vi "WFCompose.vi"(7 "Repetitions":T1 {"Interval (s)" min=0.0; "Delay (s)" min=0.0}, 8 "error in (no error)":errorcluster, 11 "Waveform In":waveform(dbl)) -> (0 "error out":errorcluster, 3 "Analog Waveform Out":waveform(dbl))   [LabVIEW 2009]
uses:
  <vilib>/Waveform/WDTOps.llb/WDT Number of Waveform Samples DBL.vi
  <vilib>/Waveform/WDTOps.llb/WDT Waveform Duration DBL.vi
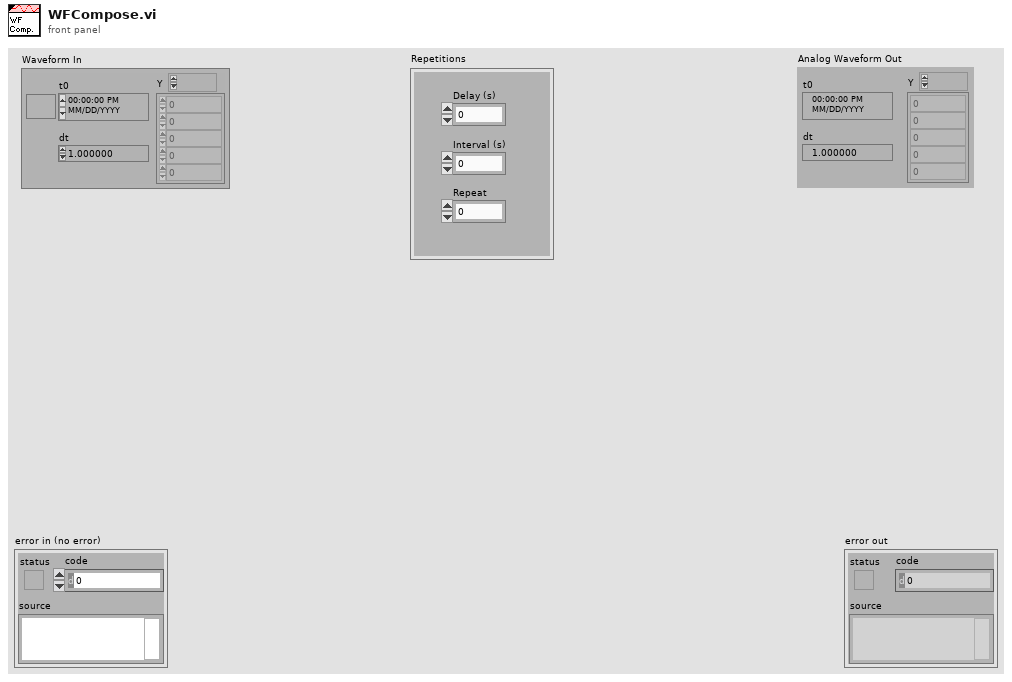
[diagram p1: front panel]
types:
  T1 = cluster{"Delay (s)":dbl, "Interval (s)":dbl, "Repeat":i32}
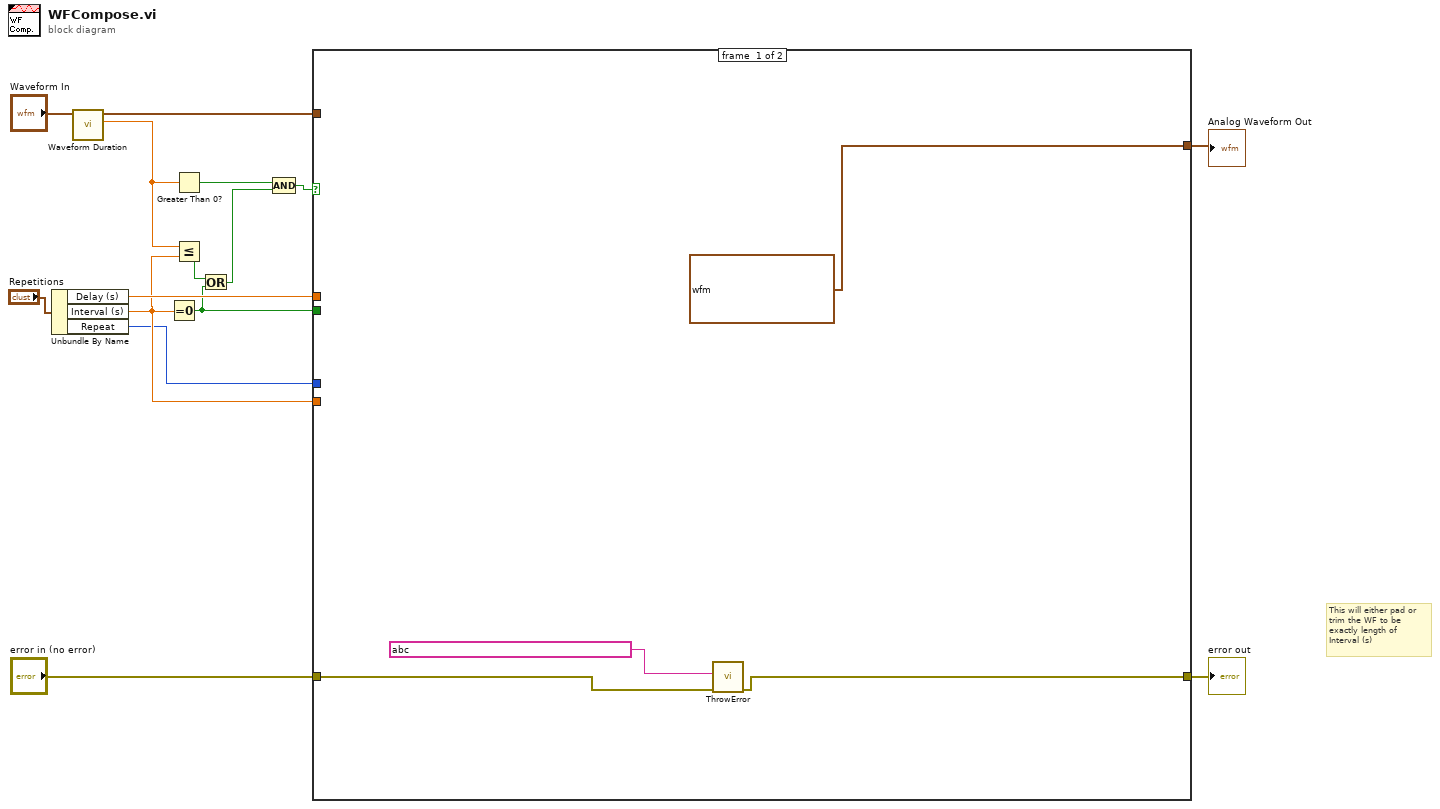
[diagram p0: block diagram]
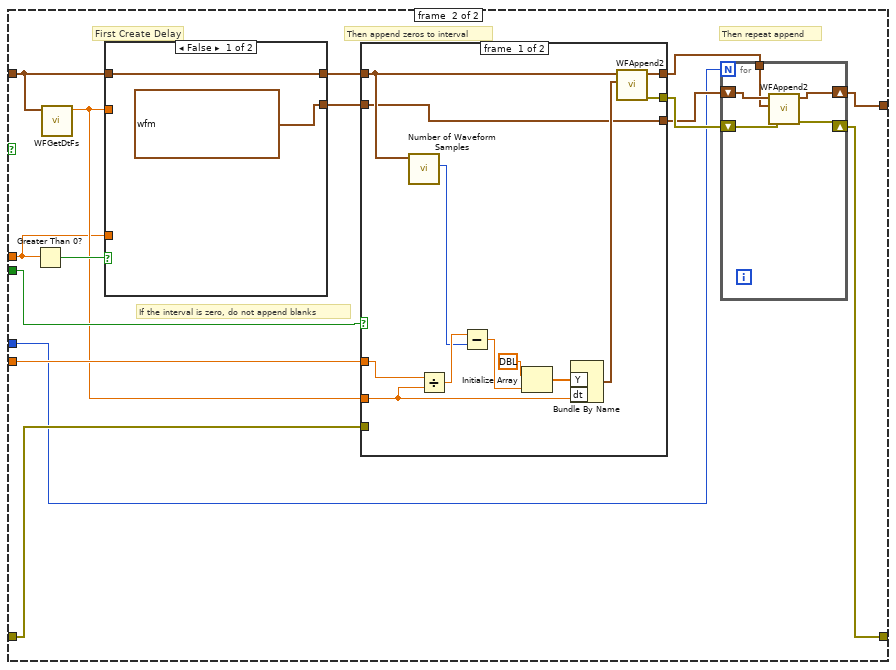
[diagram p2: hidden frame]
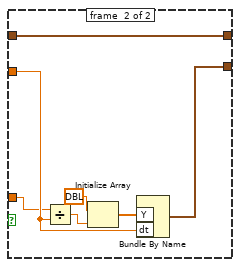
[diagram p4: hidden frame]
diagram:
  # "This will either pad or\ntrim the WF to be\nexactly length of \nInterval (s)"
  n1 = Unbundle By Name("Repetitions") -> ("Delay (s)"=w11:dbl, "Interval (s)"=w7:dbl, "Repeat"=w6:i32)
  n2 = call-poly <vilib>:"Waveform Duration.vi"("waveform in"="Waveform In") -> ("duration"=w5:dbl, "waveform out"=w2:waveform(dbl))  [unwired: 8 in, 1 out]
  n3 = Equal To 0?(x=w7) -> (x = 0?=w1:bool)
  n4 = Greater Than 0?(x=w5) -> (x > 0?=w10:bool)
  n5 = Less Or Equal?(x=w5, y=w7) -> (x <= y?=w12:bool)
  n6 = Or(x=w12, y=w1) -> (x .or. y?=w9:bool)
  n7 = Compound Arithmetic op=AND(w10, w9) -> (w8:bool)
  n8 = case shown="True" w8 {
    tunnel: "error in (no error)" -> [w18 w27]
    tunnel: w2 -> [_ w28]
    tunnel: w11 -> [_ w26]
    tunnel: w1 -> [_ w33]
    tunnel: w7 -> [_ w30]
    tunnel: w6 -> [_ w20]
    tunnel: [waveform(dbl) ? ("Waveform") w25] -> w4
    tunnel: [w17 w24] -> w3
    frame #0 {
      n9 = call "ThrowError.vi"("error in (no error)"=w18, "Error Message"=string ?) -> ("error out"=w17:errorcluster)  [unwired: 8 in, 1 out]
    }
    frame #1 {
      # "Then repeat append"
      # "If the interval is zero, do not append blanks"
      # "First Create Delay"
      # "Then append zeros to interval"
      n10 = Greater Than 0?(x=w26) -> (x > 0?=w34:bool)
      n11 = call "WFGetDtFs.vi"("Waveform"=w28) -> ("dt"=w29:dbl)  [unwired: 9 in, 1 out]
      n12 = case shown="False" w34 {
        tunnel: w28 -> [w56 w59]
        tunnel: [waveform(dbl) ? ("Waveform") w60] -> w32
        tunnel: [w56 w59] -> w31
        tunnel: w29 -> [_ w58]
        tunnel: w26 -> [_ w57]
        frame #0 {
        }
        frame #1 {
          n13 = Divide(x=w57, y=w58) -> (x/y=w61:dbl)
          n14 = Initialize Array(dbl ? ("element"), w61) -> (w63:dbl[])
          n15 = Bundle By Name("Y"=w63, "dt"=w58) -> (w60:waveform(dbl))  [unwired: 1 in]
        }
      }
      n16 = case shown="True" w33 {
        tunnel: w32 -> [w40 w53]
        tunnel: w31 -> [w44 w54]
        tunnel: w30 -> [w49 _]
        tunnel: w29 -> [w48 _]
        tunnel: w27 -> [_ w52]
        tunnel: [w42 w52] -> w23
        tunnel: [w41 w54] -> w22
        tunnel: [w40 w53] -> w21
        frame #0 {
          n17 = call-poly <vilib>:"Number of Waveform Samples.vi"("waveform in"=w44) -> ("number of samples"=w46:i32)  [unwired: 8 in, 2 out]
          n18 = Divide(x=w49, y=w48) -> (x/y=w47:dbl)
          n19 = Subtract(x=w47, y=w46) -> (x-y=w45:dbl)
          n20 = Initialize Array(dbl ? ("element"), w45) -> (w51:dbl[])
          n21 = Bundle By Name("Y"=w51, "dt"=w48) -> (w43:waveform(dbl))  [unwired: 1 in]
          n22 = call "WFAppend2.vi"("Waveform In 2"=w43, "Waveform In"=w44) -> ("error out"=w42:errorcluster, "Waveform Out"=w41:waveform(dbl))  [unwired: 4 in]
        }
        frame #1 {
          # "If interval is zero, just keep appending WF"
        }
      }
      n23 = for {
        N: w20 -> [_]
        shift-right: [w38] -> w25
        shift-left: w21 -> [w39]
        shift-right: [w36] -> w24
        shift-left: w23 -> [w37]
        tunnel: w22 -> [w35]
        n24 = call "WFAppend2.vi"("error in (no error)"=w37, "Waveform In 2"=w35, "Waveform In"=w39) -> ("error out"=w36:errorcluster, "Waveform Out"=w38:waveform(dbl))  [unwired: 3 in]
      }
    }
  }
  "error out" <- w3
  "Analog Waveform Out" <- w4
